vi "FirstOrderFilter.vi"(9 "fps":dbl, 10 "fc":dbl, 11 "Numeric in":dbl) -> (3 "Numeric out":dbl)   [LabVIEW 2018]
panel:
  out "Waveform Chart":dbl[](graph)
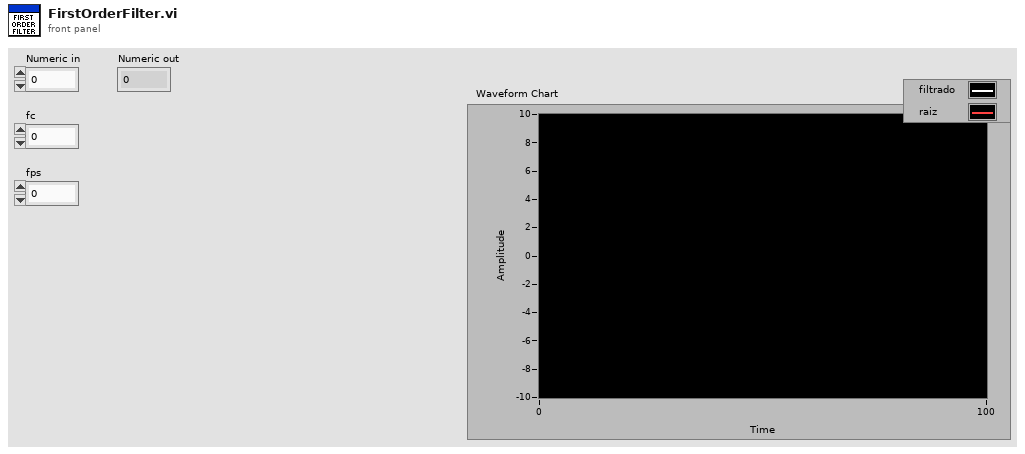
[diagram p1: front panel]
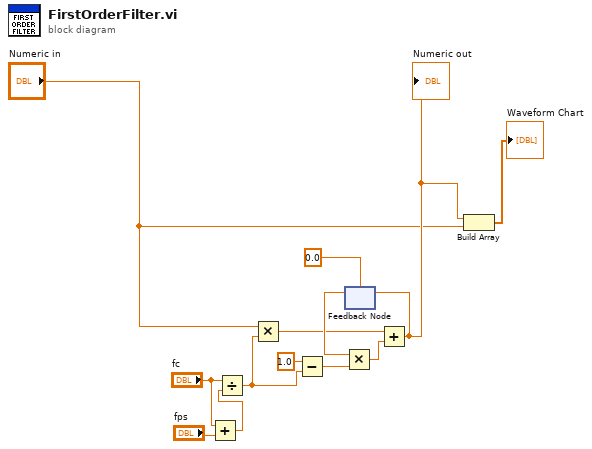
[diagram p0: block diagram]
diagram:
  n1 = Add(x="fc", y="fps") -> (x+y=w11:dbl)
  n2 = Divide(x="fc", y=w11) -> (x/y=w5:dbl)
  n3 = Multiply(x="Numeric in", y=w5) -> (x*y=w8:dbl)
  n4 = Subtract(x=1.0, y=w5) -> (x-y=w6:dbl)
  n5 = feedback #1(0.0) -> (w9:dbl)
  n6 = Multiply(x=w9, y=w6) -> (x*y=w7:dbl)
  n7 = Add(x=w8, y=w7) -> (x+y=w2:dbl)
  "Numeric out" <- w2
  n8 = feedback-in #1(w2) -> ()
  n9 = Build Array(w2, "Numeric in") -> (→"Waveform Chart":dbl[])
